vi "CTR_to_DutyCycle.vi"(2 "LOW CTR":u32, 3 "HIGH CTR":u32) -> (0 "duty cycle fraction [0-1]":dbl, 1 "period [s]":dbl)   [LabVIEW 2013]
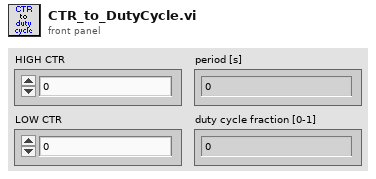
[diagram p1: front panel]
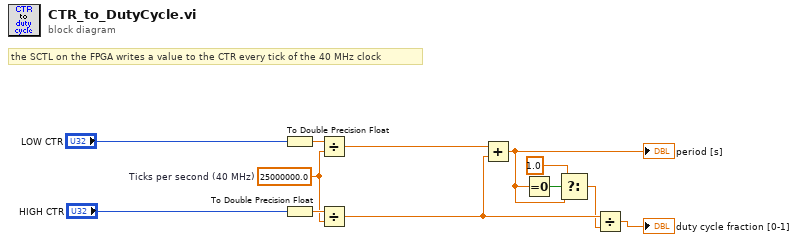
[diagram p0: block diagram]
diagram:
  w8 = 25000000.0  # Ticks per second (40 MHz)
  # "the SCTL on the FPGA writes a value to the CTR every tick of the 40 MHz clock"
  n1 = To Double Precision Float(number="LOW CTR") -> (double precision float=w9:dbl)
  n2 = To Double Precision Float(number="HIGH CTR") -> (double precision float=w10:dbl)
  n3 = Divide(x=w9, y=w8) -> (x/y=w7:dbl)
  n4 = Divide(x=w10, y=w8) -> (x/y=w6:dbl)
  n5 = Add(x=w7, y=w6) -> (x+y=w3:dbl)
  "period [s]" <- w3
  n6 = Equal To 0?(x=w3) -> (x = 0?=w4:bool)
  n7 = Select(t=1.0, s=w4, f=w3) -> (s? t:f=w2:dbl)
  n8 = Divide(x=w6, y=w2) -> (x/y=→"duty cycle fraction [0-1]":dbl)
